vi "TCP Ping(DotNET).vi"(8 "error in (no error)":errorcluster, 10 "timeout(100)":i32=100, 11 "hostName/IP Address":string="127.0.0.1") -> (0 "error out":errorcluster, 2 "Status":i32(ring) items=["Success"=0, "DestinationNetworkUnreachable"=11002, "DestinationHostUnreachable"=11003, "DestinationProhibited, DestinationProtocolUnreachable"=11004, "DestinationPortUnreachable"=11005, "NoResources"=11006, "BadOption"=11007, "HardwareError"=11008, "PacketTooBig"=11009, "TimedOut"=11010, "BadRoute"=11012, "TtlExpired"=11013, "TtlReassemblyTimeExceeded"=11014, "ParameterProblem"=11015, "SourceQuench"=11016, "BadDestination"=11018, "DestinationUnreachable"=11040, "TimeExceeded"=11041, "BadHeader"=11042, "UnrecognizedNextHeader"=11043, "IcmpError"=11044, "DestinationScopeMismatch"=11045, "Unknown"=-1])   [LabVIEW 2017]
doc: "Pings hostName/IP Address using the .NET Ping class and returns the round-trip status. The timeout(100) input is in milliseconds."
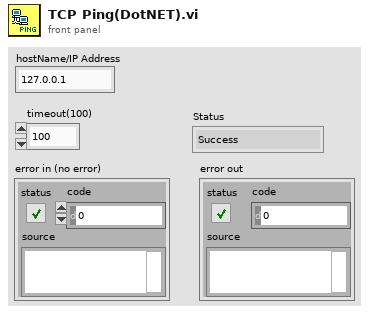
[diagram p1: front panel]
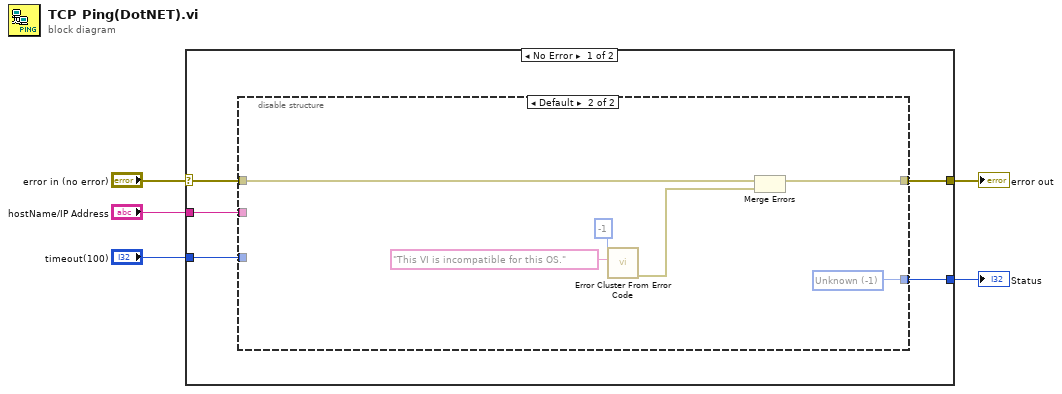
[diagram p0: block diagram]
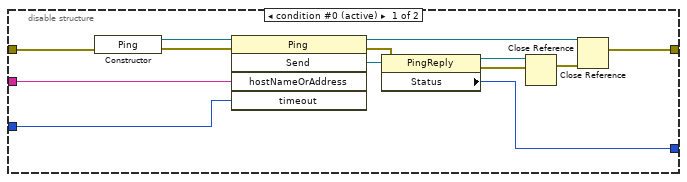
[diagram p2: hidden frame]
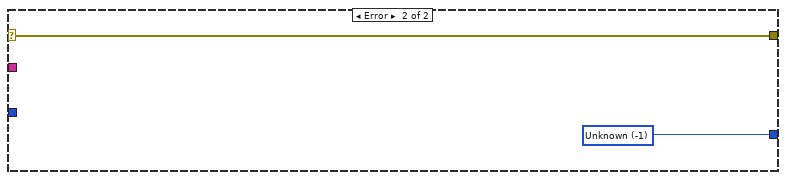
[diagram p3: hidden frame]
diagram:
  n1 = case shown="No Error" "error in (no error)" {
    selector: "error in (no error)" -> [w9 w31]
    tunnel: [w10 w31] -> w5
    tunnel: [w8 w30] -> w3
    tunnel: "hostName/IP Address" -> [w7 _]
    tunnel: "timeout(100)" -> [w6 _]
    frame No Error {
      n2 = disable-structure shown="Default" {
        disable-tunnel: [w23 w27] -> w10
        disable-tunnel: w9 -> [w22 w29]
        disable-tunnel: [w15 w28] -> w8
        disable-tunnel: w7 -> [w13 _]
        disable-tunnel: w6 -> [w11 _]
        frame condition #0 (active) {
          n3 = constructor class="Ping" ("Constructor Node")(error in=w22) -> (reference out=w14:refnum<k24>, error out=w18:errorcluster)  [unwired: 2 in, 1 out]
          n4 = invoke on="Invoke Node" class="Ping" method="Send"(reference=w14, error in=w18, "hostNameOrAddress"=w13, "timeout"=w11) -> (reference out=w17:refnum<k24>, error out=w19:errorcluster, "Send"=w12:refnum<k24>)  [unwired: 1 in, 2 out]
          n5 = property on="Property Node" class="PingReply"(reference=w12, error in=w19) -> (reference out=w16:refnum<k24>, error out=w20:errorcluster, "Status"=w15:i32)
          n6 = Close Reference(reference=w16, error in (no error)=w20) -> (error out=w21:errorcluster)
          n7 = Close Reference(reference=w17, error in (no error)=w21) -> (error out=w23:errorcluster)
        }
        frame condition #1 {
          w28 = -1 items=["Success"=0, "DestinationNetworkUnreachable"=11002, "DestinationHostUnreachable"=11003, "DestinationProhibited, DestinationProtocolUnreachable"=11004, "DestinationPortUnreachable"=11005, "NoResources"=11006, "BadOption"=11007, "HardwareError"=11008, "PacketTooBig"=11009, "TimedOut"=11010, "BadRoute"=11012, "TtlExpired"=11013, "TtlReassemblyTimeExceeded"=11014, "ParameterProblem"=11015, "SourceQuench"=11016, "BadDestination"=11018, "DestinationUnreachable"=11040, "TimeExceeded"=11041, "BadHeader"=11042, "UnrecognizedNextHeader"=11043, "IcmpError"=11044, "DestinationScopeMismatch"=11045, "Unknown"=-1] ("Status")
          n8 = call <vilib>:"Error Cluster From Error Code.vi"("error message (\"\")"="This VI is incompatible for this OS." ("error message (\"\")"), "error code (0)"=-1) -> ("error out"=w26:errorcluster)  [unwired: 7 in]
          n9 = Merge Errors(w29, w26) -> (w27:errorcluster)
        }
      }
    }
    frame Error {
      w30 = -1 items=["Success"=0, "DestinationNetworkUnreachable"=11002, "DestinationHostUnreachable"=11003, "DestinationProhibited, DestinationProtocolUnreachable"=11004, "DestinationPortUnreachable"=11005, "NoResources"=11006, "BadOption"=11007, "HardwareError"=11008, "PacketTooBig"=11009, "TimedOut"=11010, "BadRoute"=11012, "TtlExpired"=11013, "TtlReassemblyTimeExceeded"=11014, "ParameterProblem"=11015, "SourceQuench"=11016, "BadDestination"=11018, "DestinationUnreachable"=11040, "TimeExceeded"=11041, "BadHeader"=11042, "UnrecognizedNextHeader"=11043, "IcmpError"=11044, "DestinationScopeMismatch"=11045, "Unknown"=-1] ("Status")
    }
  }
  "error out" <- w5
  "Status" <- w3
